vi "Southampton_Elad.vi"(1 "Demand Voltage":dbl) -> (0 "error out":errorcluster)   [LabVIEW 2011]
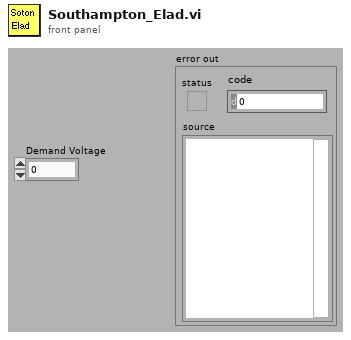
[diagram p1: front panel]
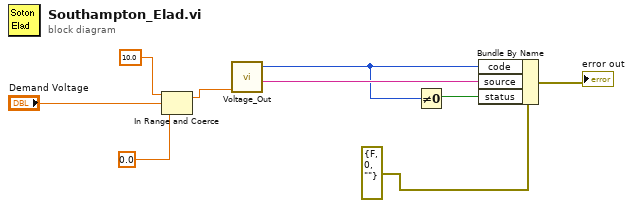
[diagram p0: block diagram]
diagram:
  n1 = In Range and Coerce(upper limit=10.0, x="Demand Voltage", lower limit=0.0) -> (coerced(x)=w3:dbl)  [unwired: 1 out]
  n2 = call "Voltage_Out.VI"("Eng Units"=w3) -> ("ErrMsg"=w8:string, "ErrCode"=w2:i32)  [unwired: 3 in]
  n3 = Not Equal To 0?(x=w2) -> (x != 0?=w1:bool)
  n4 = Bundle By Name(cluster=errorcluster {"status"=FALSE, "code"=0, "source"=""} ("error out"), "code"=w2, "source"=w8, "status"=w1) -> (→"error out":errorcluster)
